vi "CV_calc_capacitance.vi"(8 "error in (no error)":errorcluster, 9 "Theta (Phase)":dbl, 10 "Z (impedance)":dbl, 11 "Input parameters":T1={"Measurement type"=enum."Debug", "Sensor type"=enum."HPK_8in_256ch", "Identifier"="test.txt", "Open after execution?"=FALSE, "Plot after execution?"=FALSE, "Display channel"=0, "Voltage Delay (s)"=0.5, "Switch Delay (s)"=0.01, "VISA resource name source"="", "VISA resource name DMM"="", "VISA resource name LCR"="", "Compliance  Level (A)"=10.0, "Voltage Limit (V)"=1000.0, "Data storage location"="", "Scan voltages"="", "Use source as DMM?"=FALSE, "LCR signal frequenzy (Hz)"=10.0, "DMM device"=enum."Keithley2001", "Sampling number"=1, "Use env. sensors on"=enum."Sensirion sht1x/7x", "Switchboard Handle"=0, "Use Switchboard"=FALSE, "LCR signal voltage (V)"=10000.0, "Repeat"=1, "Scan voltages IV"="", "Scan voltages CV"="", "Hex pad numbers?"=FALSE, "Set measurement type"=enum."Debug", "Custom pad scan"="", "IV voltage Delay (s)"=0.5, "CV voltage Delay (s)"=0.5, "Needle measurement?"=FALSE, "Comments"="test.txt", "LCR signal frequenzy (kHz)"=10.0, "Compliance  Level (uA)"=10.0, "Open Correction Array"=array2304x3[6912 elements], "Current set voltage"=0.0, "Last set voltage"=0.0, "Current channel"=0, "Last OpenCorrection index"=-1, "Total curr/vltg every x steps"=10, "Current channel iteration"=0, "No CV corrections"=FALSE, "Mapfile"="", "Corrfile"="", "IV voltage file"=path "", "CV voltage file"=path "", "IV Switch Delay (s)"=0.01, "CV Switch Delay (s)"=0.01, "Invert polarity"=FALSE, "Set debug dirs"=FALSE, "Is n on p"=FALSE} {"CV Switch Delay (s)" format="%#_13g"; "IV Switch Delay (s)" format="%#_13g"; "Last set voltage" format="%#_13g"; "Current set voltage" format="%#_13g"; "CV voltage Delay (s)" format="%#_13g"; "IV voltage Delay (s)" format="%#_13g"; "Voltage Limit (V)" format="%#_13g"; "Voltage Delay (s)" format="%#_13g"; "Switch Delay (s)" format="%#_13g"}) -> (0 "error out":errorcluster, 1 "Cs [pF]":dbl, 2 "Cp [pF]":dbl, 3 "Input parameters out":T1={"Measurement type"=enum."Debug", "Sensor type"=enum."HPK_8in_256ch", "Identifier"="test.txt", "Open after execution?"=FALSE, "Plot after execution?"=FALSE, "Display channel"=0, "Voltage Delay (s)"=0.5, "Switch Delay (s)"=0.01, "VISA resource name source"="", "VISA resource name DMM"="", "VISA resource name LCR"="", "Compliance  Level (A)"=10.0, "Voltage Limit (V)"=1000.0, "Data storage location"="", "Scan voltages"="", "Use source as DMM?"=FALSE, "LCR signal frequenzy (Hz)"=10.0, "DMM device"=enum."Keithley2001", "Sampling number"=1, "Use env. sensors on"=enum."Sensirion sht1x/7x", "Switchboard Handle"=0, "Use Switchboard"=FALSE, "LCR signal voltage (V)"=10000.0, "Repeat"=1, "Scan voltages IV"="", "Scan voltages CV"="", "Hex pad numbers?"=FALSE, "Set measurement type"=enum."Debug", "Custom pad scan"="", "IV voltage Delay (s)"=0.5, "CV voltage Delay (s)"=0.5, "Needle measurement?"=FALSE, "Comments"="test.txt", "LCR signal frequenzy (kHz)"=10.0, "Compliance  Level (uA)"=10.0, "Open Correction Array"=array2304x3[6912 elements], "Current set voltage"=0.0, "Last set voltage"=0.0, "Current channel"=0, "Last OpenCorrection index"=-1, "Total curr/vltg every x steps"=10, "Current channel iteration"=0, "No CV corrections"=FALSE, "Mapfile"="", "Corrfile"="", "IV voltage file"=path "", "CV voltage file"=path "", "IV Switch Delay (s)"=0.01, "CV Switch Delay (s)"=0.01, "Invert polarity"=FALSE, "Set debug dirs"=FALSE, "Is n on p"=FALSE} {"CV Switch Delay (s)" format="%#_13g"; "IV Switch Delay (s)" format="%#_13g"; "Last set voltage" format="%#_13g"; "Current set voltage" format="%#_13g"; "CV voltage Delay (s)" format="%#_13g"; "IV voltage Delay (s)" format="%#_13g"; "Voltage Limit (V)" format="%#_13g"; "Voltage Delay (s)" format="%#_13g"; "Switch Delay (s)" format="%#_13g"}, 4 "Cs uncorrected [pF]":dbl, 5 "Cp uncorrected [pF]":dbl)   [LabVIEW 2016]
doc: "Determines human usable quantities from phase and impedance determined by LCR meter."
uses:
  input_params.ctl
panel:
  out "Rs [Ohm]":dbl
  out "Rp [Ohm]":dbl
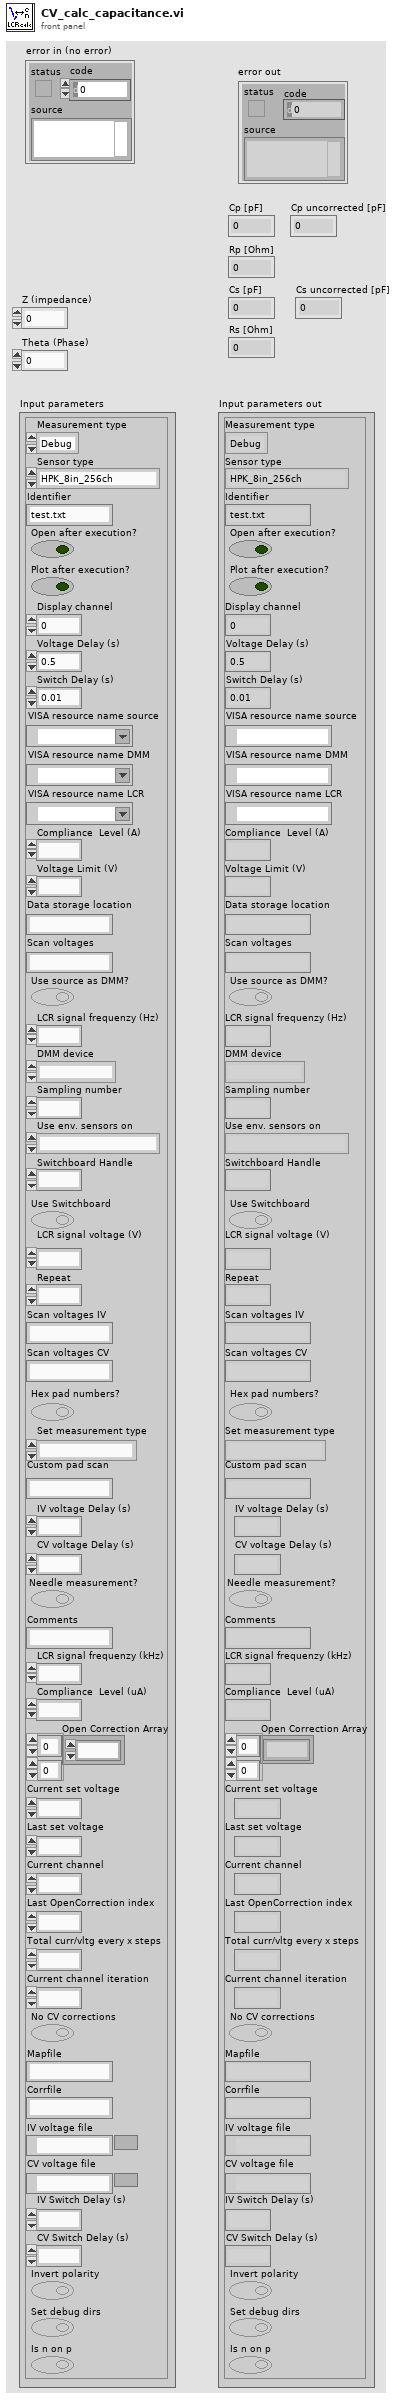
[diagram p1: front panel]
types:
  T1 = typedef "input_params.ctl" = cluster{"Measurement type":enum16{"IV", "CV", "Debug", "Test_contact"}, "Sensor type":enum16{"HPK_6in_135ch", "HPK_8in_256ch", "IFX_8in_256ch", "Diode", "HPK_6in_256ch", "Full_Matrix", ""}, "Identifier":string, "Open after execution?":bool, "Plot after execution?":bool, "Display channel":i32, "Voltage Delay (s)":dbl, "Switch Delay (s)":dbl, "VISA resource name source":refnum<visa-resource-name>, "VISA resource name DMM":refnum<visa-resource-name>, "VISA resource name LCR":refnum<visa-resource-name>, "Compliance  Level (A)":dbl, "Voltage Limit (V)":dbl, "Data storage location":string, "Scan voltages":string, "Use source as DMM?":bool, "LCR signal frequenzy (Hz)":dbl, "DMM device":enum16{"Keithley2001", "Keithley2450", "Keithley2410", "Keithley6487", "Keithley6514"}, "Sampling number":i32, "Use env. sensors on":enum16{"Sensirion sht1x/7x", "Switch Matrix", "Probecard"}, "Switchboard Handle":u32, "Use Switchboard":bool, "LCR signal voltage (V)":dbl, "Repeat":i32, "Scan voltages IV":string, "Scan voltages CV":string, "Hex pad numbers?":bool, "Set measurement type":enum16{"IV", "CV", "Debug", "Test_contact", "IV+CV"}, "Custom pad scan":string, "IV voltage Delay (s)":dbl, "CV voltage Delay (s)":dbl, "Needle measurement?":bool, "Comments":string, "LCR signal frequenzy (kHz)":dbl, "Compliance  Level (uA)":dbl, "Open Correction Array":dbl[][], "Current set voltage":dbl, "Last set voltage":dbl, "Current channel":i32, "Last OpenCorrection index":i32, "Total curr/vltg every x steps":i32, "Current channel iteration":i32, "No CV corrections":bool, "Mapfile":string, "Corrfile":string, "IV voltage file":path, "CV voltage file":path, "IV Switch Delay (s)":dbl, "CV Switch Delay (s)":dbl, "Invert polarity":bool, "Set debug dirs":bool, "Is n on p":bool}
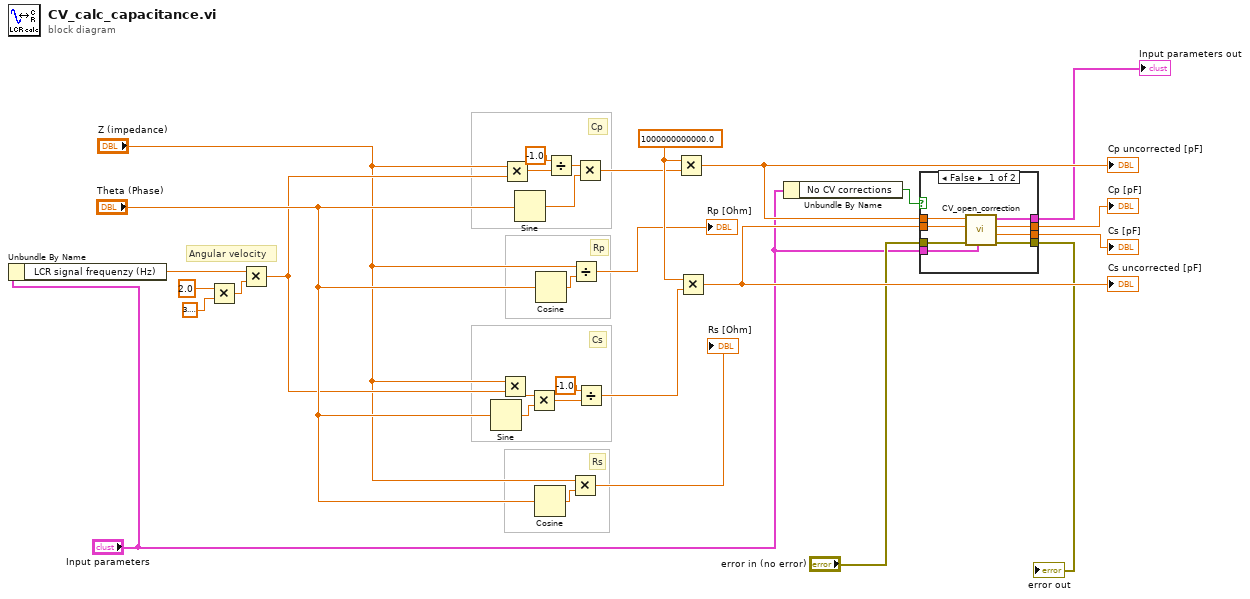
[diagram p0: block diagram]
diagram:
  w31 = 1000000000000.0 ("y")
  # "Cp"
  # "Angular velocity"
  # "Rp"
  # "Cs"
  # "Rs"
  n1 = Unbundle By Name("Input parameters") -> ("LCR signal frequenzy (Hz)"=w3:dbl)
  n2 = Multiply(x=2.0, y=3.141592653589793) -> (x*y=w25:dbl)
  n3 = Multiply(x=w3, y=w25) -> (x*y=w13:dbl)
  n4 = Sine(x="Theta (Phase)") -> (sin(x)=w23:dbl)
  n5 = Multiply(x="Z (impedance)", y=w13) -> (x*y=w24:dbl)
  n6 = Multiply(x="Z (impedance)", y=w13) -> (x*y=w14:dbl)
  n7 = Sine(x="Theta (Phase)") -> (sin(x)=w16:dbl)
  n8 = Multiply(x=w24, y=w23) -> (x*y=w22:dbl)
  n9 = Cosine(x="Theta (Phase)") -> (cos(x)=w30:dbl)
  n10 = Cosine(x="Theta (Phase)") -> (cos(x)=w20:dbl)
  n11 = Divide(x=-1.0, y=w14) -> (x/y=w17:dbl)
  n12 = Multiply(x="Z (impedance)", y=w30) -> (x*y=→"Rs [Ohm]":dbl)
  n13 = Divide(x="Z (impedance)", y=w20) -> (x/y=→"Rp [Ohm]":dbl)
  n14 = Multiply(x=w17, y=w16) -> (x*y=w11:dbl)
  n15 = Divide(x=-1.0, y=w22) -> (x/y=w21:dbl)
  n16 = Multiply(x=w31, y=w11) -> (x*y=w10:dbl)
  "Cp uncorrected [pF]" <- w10
  n17 = Multiply(x=w31, y=w21) -> (x*y=w9:dbl)
  "Cs uncorrected [pF]" <- w9
  n18 = Unbundle By Name("Input parameters") -> ("No CV corrections"=w1:bool)
  n19 = case shown="False" w1 {
    tunnel: w10 -> [w39 w43]
    tunnel: w9 -> [w38 w42]
    tunnel: "error in (no error)" -> [w37 w40]
    tunnel: [w36 w40] -> w7
    tunnel: [w35 w42] -> w6
    tunnel: [w34 w43] -> w5
    tunnel: [w33 w41] -> w4
    tunnel: "Input parameters" -> [w32 w41]
    frame False {
      n20 = call "CV_open_correction.vi"("Input parameters"=w32, "error in (no error)"=w37, "Cs [pF]"=w38, "Cp [pF]"=w39) -> ("error out"=w36:errorcluster, "Cs corrected [pF]"=w35:dbl, "Cp corrected [pF]"=w34:dbl, "Input parameters out"=w33:T1)  [unwired: 4 in]
    }
    frame True {
    }
  }
  "Cp [pF]" <- w5
  "Cs [pF]" <- w6
  "error out" <- w7
  "Input parameters out" <- w4
